vi "CMD_Shoot.vi"(1 "Line":string) -> (0 "Done":bool)   [LabVIEW 2015]
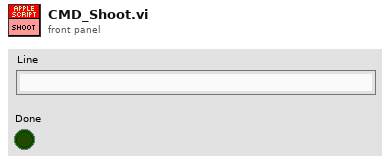
[diagram p1: front panel]
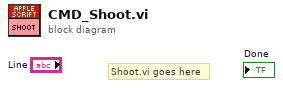
[diagram p0: block diagram]
diagram:
  # "Shoot.vi goes here"
